vi "Read Device ID Laser.vi"(8 "error in (no error)":errorcluster, 11 "NKT in":refnum<class "NKT_Extreme.lvclass">) -> (0 "error out":errorcluster, 2 "Device ID Laser":u8, 3 "NKT out":refnum<class "NKT_Extreme.lvclass">)   [LabVIEW 2020, in "NKT_Extreme.lvclass"]
uses:
  <instrlib>/Classes/Laser/NKT/NKT_Extreme.lvclass
  <instrlib>/Classes/Laser/NKT/NKT_Extreme.lvclass/NKT_Extreme.ctl
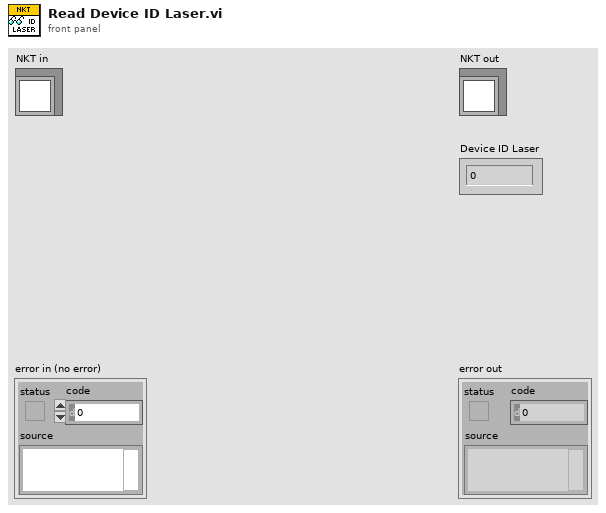
[diagram p1: front panel]
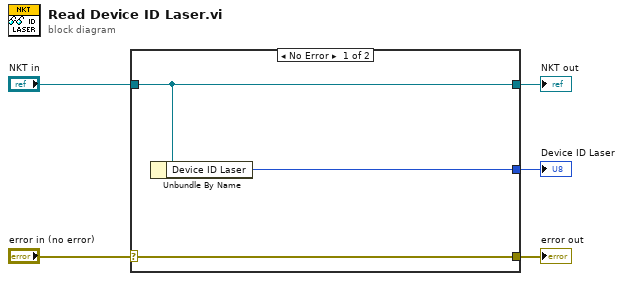
[diagram p0: block diagram]
diagram:
  n1 = case shown="No Error" "error in (no error)" {
    selector: "error in (no error)" -> [w8 w9]
    tunnel: [w8 w9] -> w4
    tunnel: [w7 w10] -> w2
    tunnel: "NKT in" -> [w7 w10]
    tunnel: [w6 _] -> w1
    frame No Error {
      n2 = Unbundle By Name(w7) -> ("Device ID Laser"=w6:u8)
    }
    frame Error {
    }
  }
  "error out" <- w4
  "NKT out" <- w2
  "Device ID Laser" <- w1
